vi "Multiply.vi"(8 "error in (no error)":errorcluster, 10 "High Res Arithmetic 2":refnum<class "Rational Number.lvclass">, 11 "High Res Arithmetic 1":refnum<class "Rational Number.lvclass">) -> (0 "error out":errorcluster, 3 "High Res Arithmetic sum":refnum<class "Rational Number.lvclass">)   [LabVIEW 2021, in "Rational Number.lvclass"]
uses:
  Rational Number.lvclass
  Rational Number.lvclass/Rational Number.ctl
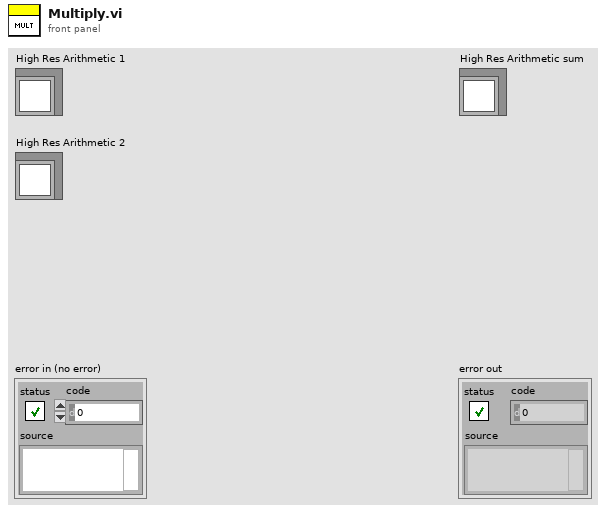
[diagram p1: front panel]
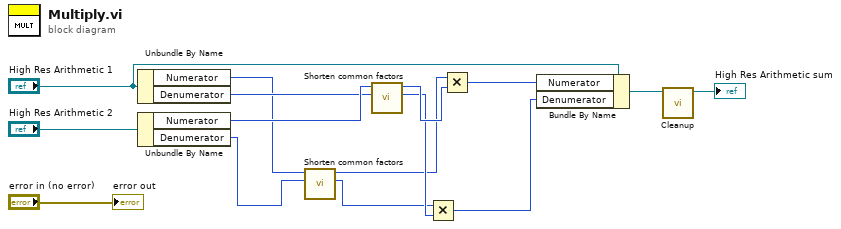
[diagram p0: block diagram]
diagram:
  n1 = Unbundle By Name("High Res Arithmetic 1") -> ("Numerator"=w4:i64, "Denumerator"=w6:i64)
  n2 = Unbundle By Name("High Res Arithmetic 2") -> ("Numerator"=w8:i64, "Denumerator"=w2:i64)
  n3 = call "Shorten common factors.vi"("Denumerator in"=w2, "Numerator in"=w4) -> ("Denumerator out"=w1:i64, "Numerator out"=w3:i64)  [unwired: 8 in]
  n4 = call "Shorten common factors.vi"("Denumerator in"=w6, "Numerator in"=w8) -> ("Denumerator out"=w5:i64, "Numerator out"=w7:i64)  [unwired: 8 in]
  n5 = Multiply(x=w1, y=w5) -> (x*y=w10:i64)
  n6 = Multiply(x=w3, y=w7) -> (x*y=w11:i64)
  n7 = Bundle By Name(cluster="High Res Arithmetic 1", "Numerator"=w11, "Denumerator"=w10) -> (w12:refnum<class "Rational Number.lvclass">)
  n8 = call "Cleanup.vi"("High Res Arithmetic in"=w12) -> ("High Res Arithmetic out"=→"High Res Arithmetic sum":refnum<class "Rational Number.lvclass">)  [unwired: 9 in, 1 out]
  "error out" <- "error in (no error)"
